vi "Test_issueCommand_setScalars.vi"(8 "error in (no error)":errorcluster, 11 "command_setScalars_Ctl":T1={"private_rcvStamp"=0.0, "boolean0"=FALSE, "byte0"=0, "char0"="", "short0"=0, "int0"=0, "long0"=0, "longLong0"=0, "octet0"=0, "unsignedShort0"=0, "unsignedInt0"=0, "unsignedLong0"=0, "float0"=0.0, "double0"=0.0, "string0"="                    "}) -> (0 "error out":errorcluster, 2 "function return":i32, 3 "command_setScalars_Ctl out":T1={"private_rcvStamp"=0.0, "boolean0"=FALSE, "byte0"=0, "char0"="", "short0"=0, "int0"=0, "long0"=0, "longLong0"=0, "octet0"=0, "unsignedShort0"=0, "unsignedInt0"=0, "unsignedLong0"=0, "float0"=0.0, "double0"=0.0, "string0"="                    "})   [LabVIEW 2018, in "SALLV_Test.lvlib"]
doc: "int Test_shm_issueCommand_setScalarsLV(Test_command_setScalarsLV *command_setScalars_Ctl );"
uses:
  DataTypes/command_setScalars.ctl
  SALLV_Test.lvlib
  SALLV_Test.so
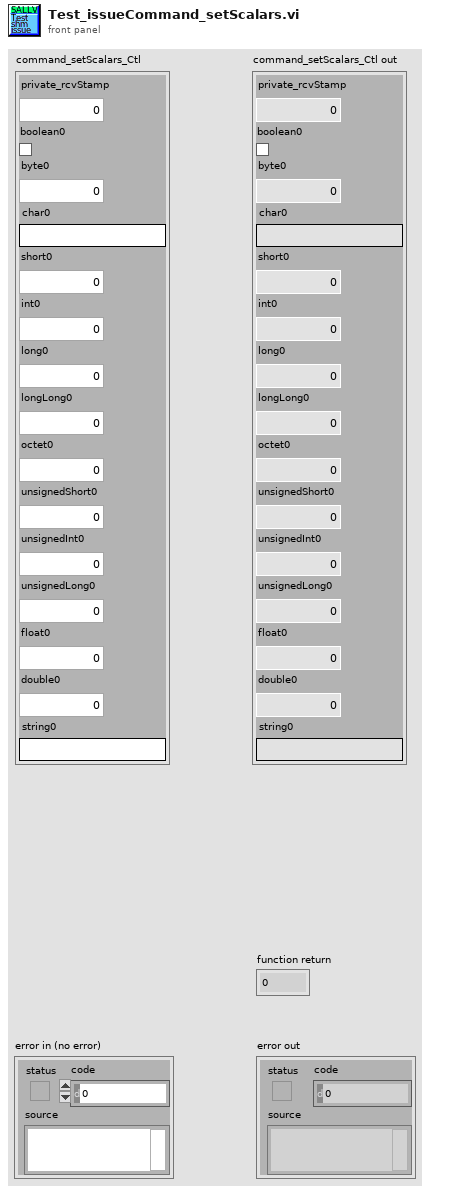
[diagram p1: front panel]
types:
  T1 = typedef "SALLV_Test.lvlib/command_setScalars.ctl" = cluster{"private_rcvStamp":dbl, "boolean0":bool, "byte0":u8, "char0":string, "short0":i16, "int0":i32, "long0":i32, "longLong0":i64, "octet0":u8, "unsignedShort0":u16, "unsignedInt0":u32, "unsignedLong0":u32, "float0":sgl, "double0":dbl, "string0":string}
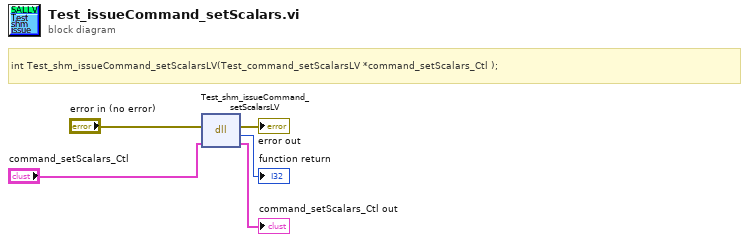
[diagram p0: block diagram]
diagram:
  # "int Test_shm_issueCommand_setScalarsLV(Test_command_setScalarsLV *command_setScalars_Ctl );"
  n1 = dll-call lib="home/ttsai/Documents/salTestLabViewApi/SALLV_Test/SALLV_Test.*" fn="Test_shm_issueCommand_setScalarsLV"(error in="error in (no error)", "command_setScalars_Ctl"="command_setScalars_Ctl") -> (error out=→"error out":errorcluster, →"function return":i32, "command_setScalars_Ctl"=→"command_setScalars_Ctl out":T1)  [unwired: 2 in, 1 out]
